vi "read-multiple-registers.vi"(8 "error in":errorcluster, 9 "id":u16, 10 "regs":u16[](array[numeric]), 11 "TCP master in":refnum<class "Modbus Master.lvclass">) -> (0 "error out":errorcluster, 2 "reading":cluster{"address":u16, "value":u16}[](array[cluster]), 3 "Modbus master out":refnum<class "Modbus Master.lvclass">)   [LabVIEW 2021]
uses:
  <vilib>/Modbus/master/Modbus Master.lvclass
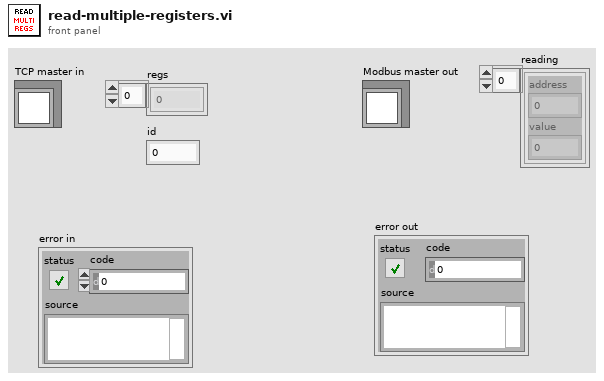
[diagram p1: front panel]
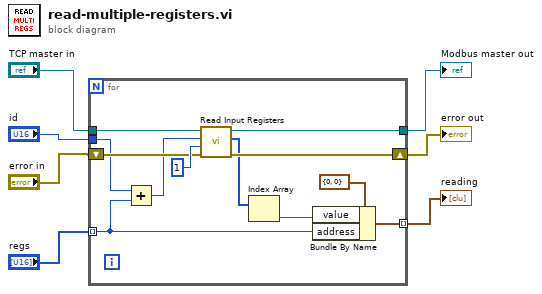
[diagram p0: block diagram]
diagram:
  n1 = for {
    tunnel: "regs" -> [w9] mode=indexing
    tunnel: "TCP master in" -> [w18]
    tunnel: [w17] -> w3
    shift-right: [w16] -> w2
    shift-left: "error in" -> [w15]
    tunnel: [w11] -> w4 mode=indexing
    tunnel: "id" -> [w10]
    n2 = Add(x=w10, y=w9) -> (x+y=w8:u16)
    n3 = call-dynamic "Read Input Registers.vi"("error in (no error)"=w15, "number of input registers"=u16 1, "starting address"=w8, "Modbus master in"=w18) -> ("error out"=w16:errorcluster, "register values"=w14:u16[], "Modbus master out"=w17:refnum<class "Modbus Master.lvclass">)  [unwired: 5 in]
    n4 = Index Array(array=w14) -> (element=w12:u16)  [unwired: 1 in]
    n5 = Bundle By Name(cluster=cluster{"address":u16, "value":u16} {"address"=0, "value"=0} ("register"), "value"=w12, "address"=w9) -> (w11:cluster{"address":u16, "value":u16})
  }
  "reading" <- w4
  "Modbus master out" <- w3
  "error out" <- w2
